vi "esp32_connection.vi"() -> ()   [LabVIEW 2020]
uses:
  <vilib>/measure/NI_MABase.lvlib
panel:
  out "Waveform Chart":waveform(dbl)(graph)
  out "?":bool
  out "Waveform Graph":waveform(dbl)(graph)
  out "Position":string
  in  "Radio Buttons":enum32{"Open", "Closed"}(radio)
  in  "Combo Box":string(combo)
  out "Output":string
  in  "?":bool
  in  "IP Address":string
  # "Connection with ESP32 through TCP"
  # "Note: Radio buttons will \nnot work in automatic mode."
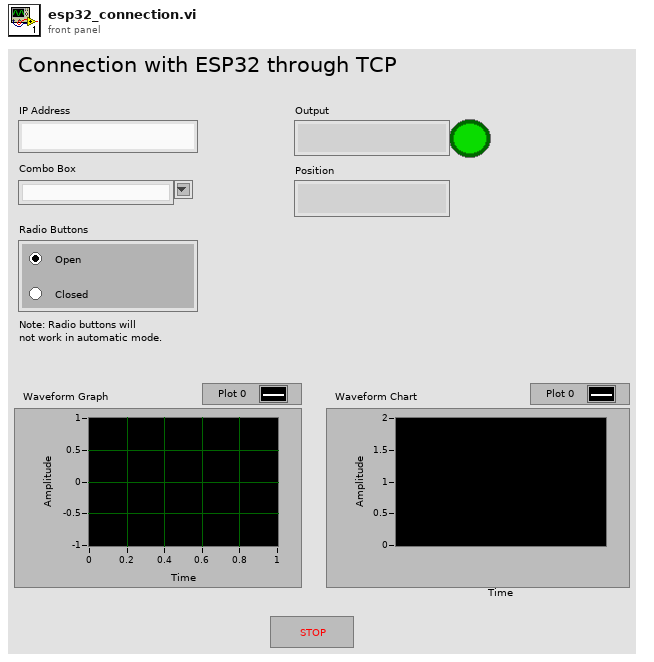
[diagram p1: front panel]
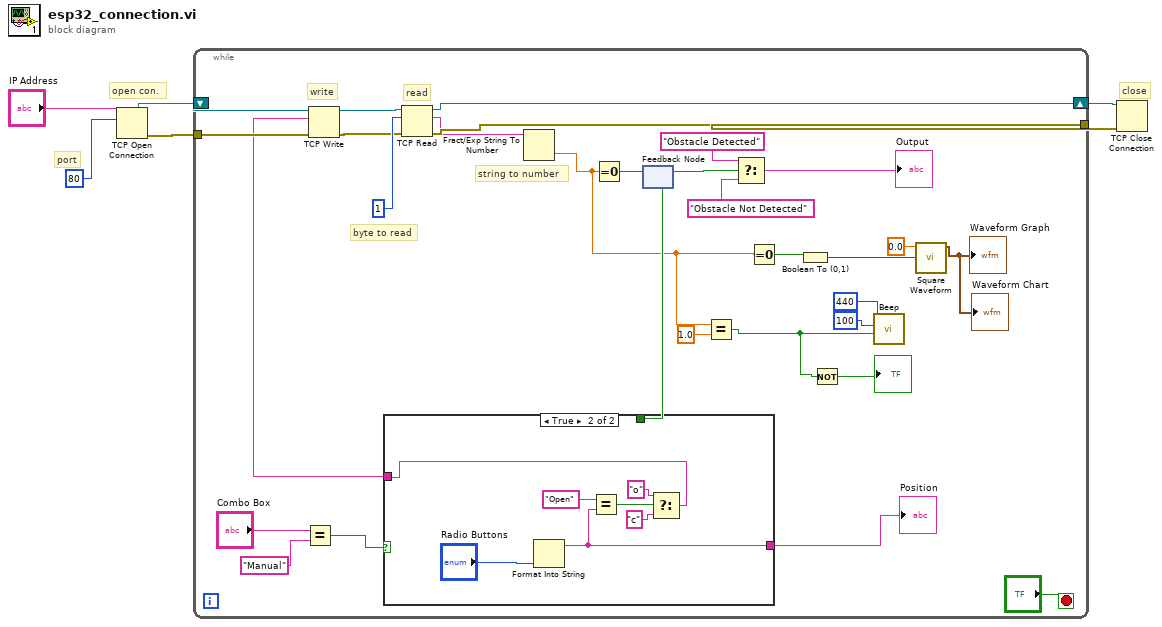
[diagram p0: block diagram]
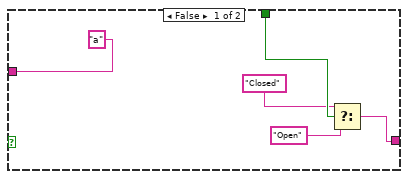
[diagram p2: hidden frame]
diagram:
  # "port"
  # "close"
  # "open con."
  n1 = TCP Open Connection(address="IP Address", remote port or service name=u16 80) -> (connection ID=w4:refnum<k5>, error out=w2:errorcluster)  [unwired: 3 in]
  n2 = while {
    shift-right: [w35] -> w3
    shift-left: w4 -> [w30]
    tunnel: w2 -> [w28]
    tunnel: [w33] -> w1
    stop <- "?" stop-if-true
    # "string to number"
    # "byte to read"
    # "read"
    # "write"
    n3 = Equal?(x="Combo Box", y="Manual") -> (x = y?=w22:bool)
    n4 = feedback #1() -> (w17:bool)  [unwired: 1 in]
    n5 = case shown="True" w22 {
      tunnel: ["a" ("y") w44] -> w21
      tunnel: [w36 w41] -> w19
      tunnel: w17 -> [w38 _]
      frame False {
        n6 = Select(t="Closed", s=w38, f="Open") -> (s? t:f=w36:string)
      }
      frame True {
        n7 = Format Into String "Format Into String"("Radio Buttons") -> (resulting string=w41:string)  [unwired: 3 in, 1 out]
        n8 = Equal?(x="Open", y=w41) -> (x = y?=w45:bool)
        n9 = Select(t="o", s=w45, f="c") -> (s? t:f=w44:string)
      }
    }
    "Position" <- w19
    n10 = TCP Write(connection ID=w30, data in=w21, error in (no error)=w28) -> (connection ID out=w29:refnum<k5>, error out=w27:errorcluster)  [unwired: 1 in, 1 out]
    n11 = TCP Read(connection ID=w29, bytes to read=1, error in (no error)=w27) -> (connection ID out=w35:refnum<k5>, data out=w31:string, error out=w33:errorcluster)  [unwired: 2 in]
    n12 = Fract/Exp String To Number(string=w31) -> (number=w10:dbl)  [unwired: 3 in, 1 out]
    n13 = Equal To 0?(x=w10) -> (x = 0?=w18:bool)
    n14 = feedback-in #1(w18) -> ()
    n15 = Equal?(x=w10, y=1.0) -> (x = y?=w12:bool)
    n16 = Select(t="Obstacle Detected", s=w17, f="Obstacle Not Detected") -> (s? t:f=→"Output":string)
    n17 = Equal To 0?(x=w10) -> (x = 0?=w9:bool)
    n18 = Boolean To (0,1)(Boolean=w9) -> (0, 1=w8:i16)
    n19 = Not(x=w12) -> (.not. x?=→"?":bool)
    n20 = call <vilib>:"Beep.vi"("use system alert? (T)"=w12, "duration (msec)"=u32 100, "frequency (Hz)"=u32 440) -> ()  [unwired: 9 in]
    n21 = call <vilib>:"Square Waveform.vi"("amplitude"=w8, "frequency"=0.0) -> ("signal out"=→"Waveform Graph" →"Waveform Chart":waveform(dbl))  [unwired: 8 in, 1 out]
  }
  n22 = TCP Close Connection(connection ID=w3, error in (no error)=w1) -> ()  [unwired: 1 in, 2 out]
